vi "disassemble_command.vi"(5 "stop byte":string="w", 7 "start byte":string="Ý", 8 "expected checksum":u16=1134, 9 "expected size of data":u8, 10 "received from serial":string="Ý¥\u0003\u000f\u0001\u0010h\r¬\r¬\u0000d\u0000d\tÄ\u0006Ö\u0004nw", 11 "command code enum":T1) -> (0 "tests":bool, 3 "data":string)   [LabVIEW 2019]
uses:
  typedefs/command.ctl
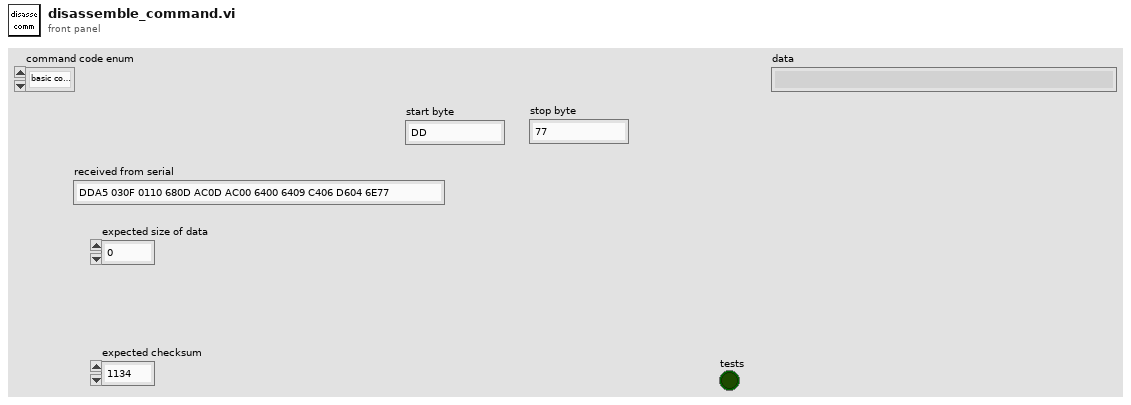
[diagram p1: front panel]
types:
  T1 = typedef "command.ctl" = enum16{"basic configuration", "test configuration", "converter configuration", "reset", "start", "next cell", "next state"}
  T2 = enum16{"big-endian, network order", "native, host order", "little-endian"}
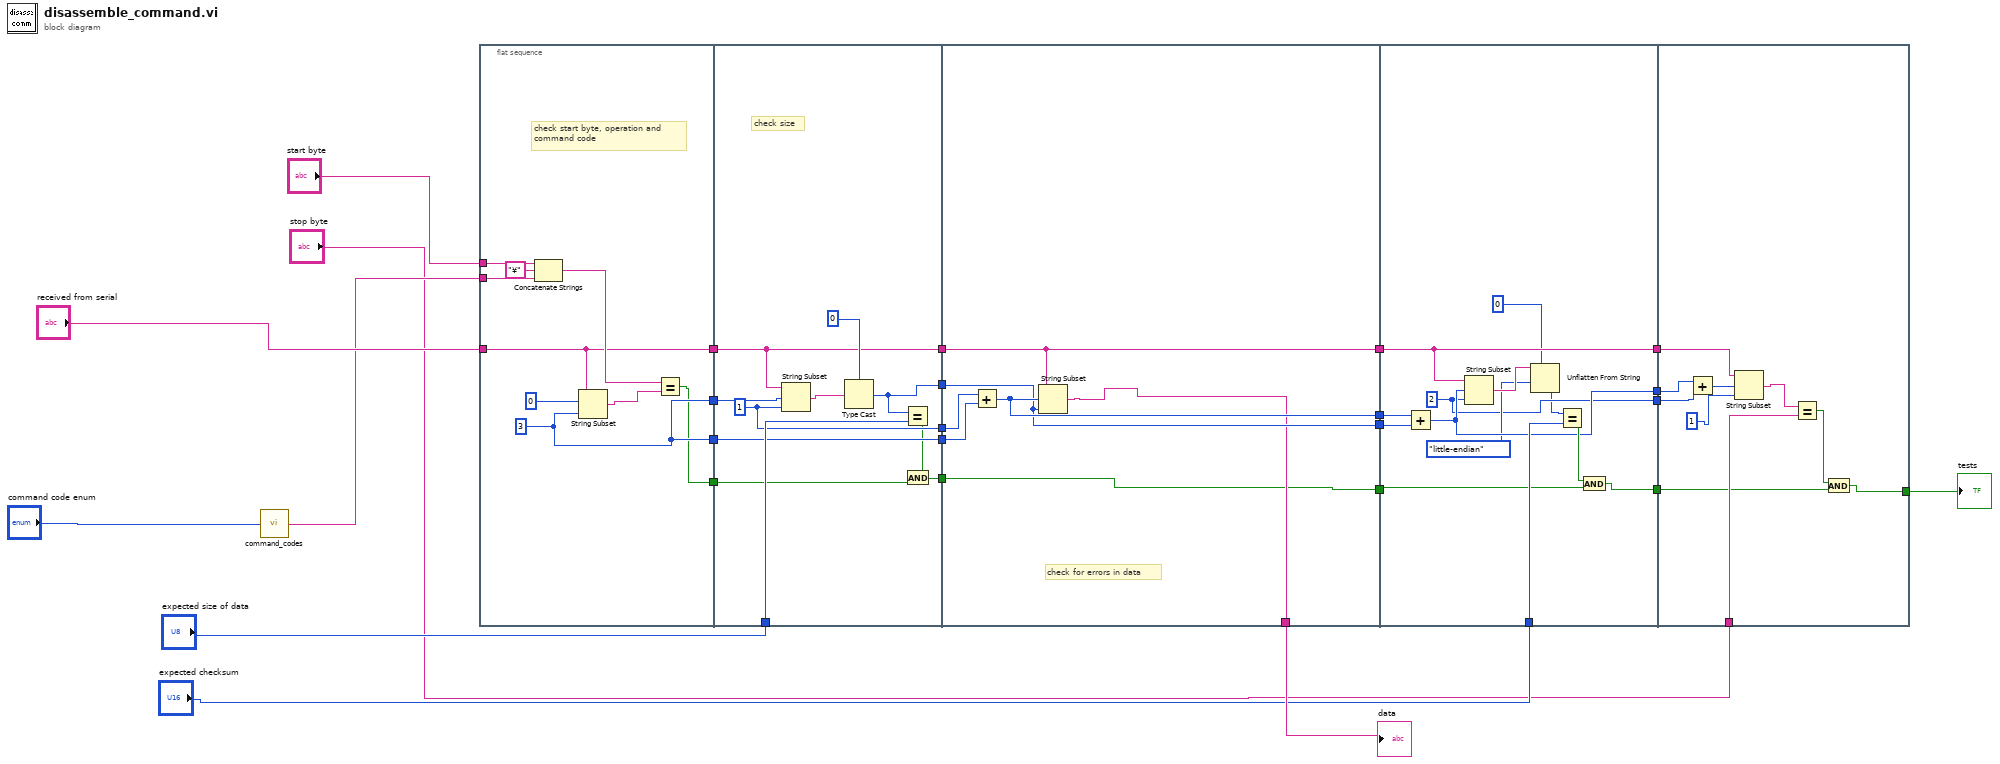
[diagram p0: block diagram]
diagram:
  n1 = call "command_codes.vi"("command code enum"="command code enum") -> ("command code"=w17:string)
  n2 = flat-sequence {
    tunnel: "received from serial" -> [w29]
    tunnel: "start byte" -> [w35]
    tunnel: w17 -> [w33]
    tunnel: [w28] -> w24
    tunnel: [w29] -> w23
    tunnel: [w28] -> w20
    tunnel: [w27] -> w15
    tunnel: w24 -> [w46]
    tunnel: w23 -> [w40]
    tunnel: "expected size of data" -> [w43]
    tunnel: [w42] -> w21
    tunnel: w20 -> [w41]
    tunnel: [w41] -> w19
    tunnel: [w36] -> w18
    tunnel: [w40] -> w16
    tunnel: w15 -> [w38]
    tunnel: [w37] -> w14
    tunnel: w21 -> [w53]
    tunnel: w19 -> [w52]
    tunnel: w18 -> [w50]
    tunnel: w16 -> [w49]
    tunnel: w14 -> [w47]
    tunnel: [w48] -> w13
    tunnel: [w47] -> w12
    tunnel: [w51] -> w11
    tunnel: [w50] -> w10
    tunnel: [w49] -> w9
    tunnel: w12 -> [w61]
    tunnel: w11 -> [w66]
    tunnel: w10 -> [w65]
    tunnel: w9 -> [w59]
    tunnel: "expected checksum" -> [w64]
    tunnel: [w63] -> w7
    tunnel: [w60] -> w6
    tunnel: [w55] -> w5
    tunnel: [w59] -> w4
    tunnel: w7 -> [w71]
    tunnel: w6 -> [w76]
    tunnel: w5 -> [w75]
    tunnel: w4 -> [w74]
    tunnel: "stop byte" -> [w72]
    tunnel: [w69] -> w2
    frame #0 {
      w28 = u8 3 ("length (rest)")
      # "check start byte, operation and\ncommand code"
      n3 = Concatenate Strings(w35, "¥" ("string"), w33) -> (w31:string)
      n4 = String Subset(string=w29, offset (0)=u8 0, length (rest)=w28) -> (substring=w32:string)
      n5 = Equal?(x=w31, y=w32) -> (x = y?=w27:bool)
    }
    frame #1 {
      w42 = u8 1 ("length (rest)")
      # "check size"
      n6 = String Subset(string=w40, offset (0)=w46, length (rest)=w42) -> (substring=w45:string)
      n7 = Type Cast(type=u8 0 ("length (rest)"), x=w45) -> (*(type *) &x=w36:u8)
      n8 = Equal?(x=w36, y=w43) -> (x = y?=w39:bool)
      n9 = And(x=w39, y=w38) -> (x .and. y?=w37:bool)
    }
    frame #2 {
      # "check for errors in data"
      n10 = Add(x=w53, y=w52) -> (x+y=w51:u8)
      n11 = String Subset(string=w49, offset (0)=w51, length (rest)=w50) -> (substring=w48:string)
    }
    frame #3 {
      w55 = u8 2 ("length (rest)")
      n12 = Add(x=w66, y=w65) -> (x+y=w60:u8)
      n13 = String Subset(string=w59, offset (0)=w60, length (rest)=w55) -> (substring=w58:string)
      n14 = Unflatten From String(type=u16 0, binary string=w58, byte order (0:big-endian, network order)=T2."little-endian") -> (value=w54:u16)  [unwired: 2 in, 2 out]
      n15 = Equal?(x=w54, y=w64) -> (x = y?=w62:bool)
      n16 = And(x=w62, y=w61) -> (x .and. y?=w63:bool)
    }
    frame #4 {
      n17 = Add(x=w76, y=w75) -> (x+y=w68:u8)
      n18 = String Subset(string=w74, offset (0)=w68, length (rest)=u8 1 ("offset (0)")) -> (substring=w73:string)
      n19 = Equal?(x=w73, y=w72) -> (x = y?=w70:bool)
      n20 = And(x=w70, y=w71) -> (x .and. y?=w69:bool)
    }
  }
  "tests" <- w2
  "data" <- w13
